vi "PHY-2019-038 (2).vi"() -> ()   [LabVIEW 2022 SP3]
panel:
  out "Message":string
  out "warnimg":bool
  out "Seconds":dbl
  out "Minutes":dbl
  out "Hours":dbl
  in  "Total time in seconds":dbl
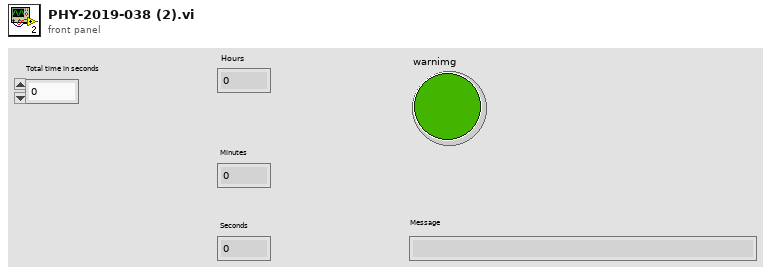
[diagram p1: front panel]
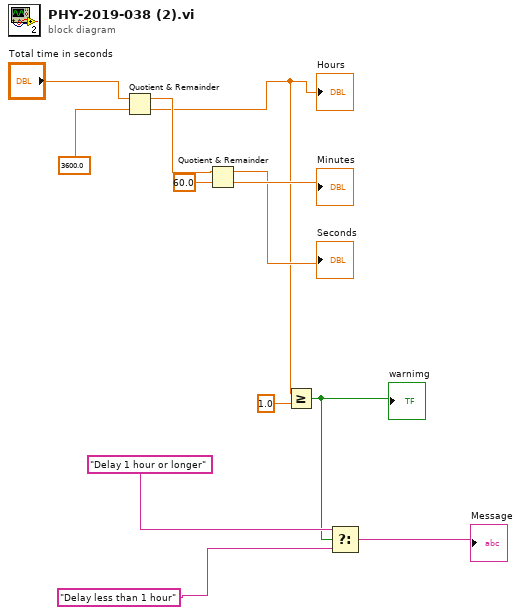
[diagram p0: block diagram]
diagram:
  n1 = Quotient & Remainder(x="Total time in seconds", y=3600.0) -> (x-y*floor(x/y)=w9:dbl, floor(x/y)=w6:dbl)
  "Hours" <- w6
  n2 = Quotient & Remainder(x=w9, y=60.0) -> (x-y*floor(x/y)=→"Seconds":dbl, floor(x/y)=→"Minutes":dbl)
  n3 = Greater Or Equal?(x=w6, y=1.0) -> (x >= y?=w3:bool)
  "warnimg" <- w3
  n4 = Select(t="Delay 1 hour or longer", s=w3, f="Delay less than 1 hour") -> (s? t:f=→"Message":string)
